vi "Set Next Round.vi"(10 "Next Round":u32, 11 "Square in":refnum<class "Square.lvclass">) -> (3 "Square out":refnum<class "Square.lvclass">)   [LabVIEW 2020, in "SquareBattle.lvlib" / "Square.lvclass"]
uses:
  Square.lvclass
  Square.lvclass/Square.ctl
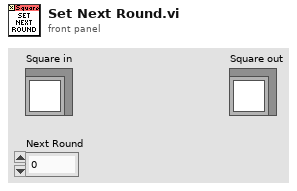
[diagram p1: front panel]
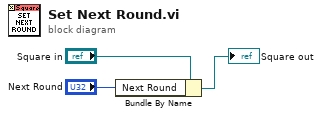
[diagram p0: block diagram]
diagram:
  n1 = Bundle By Name(cluster="Square in", "Next Round"="Next Round") -> (→"Square out":refnum<class "Square.lvclass">)
